vi "Setup.vi"(8 "error in (no error)":errorcluster, 11 "Mock Process Test In":refnum<class "Mock Process Test.lvclass">) -> (0 "error out":errorcluster, 3 "Mock Process Test Out":refnum<class "Mock Process Test.lvclass">)   [LabVIEW 2020, in "Mock Process Test.lvclass"]
uses:
  Base Class Test/Base Test.lvclass/Base Test.ctl
  Mock Process Test.lvclass
  Base Class Test/Base Test.lvclass
  Mock Process/Mock Process.lvclass
  C:/Users/anton/Documents/GitHub/Triarc-Framework/source/Framework/Process/Process.lvclass
  C:/Users/anton/Documents/GitHub/Triarc-Framework/source/Framework/Base/Base.lvclass
  C:/Users/anton/Documents/GitHub/Triarc-Framework/source/Framework/Error Handler Interface/Error Handler Interface.lvclass
  C:/Users/anton/Documents/GitHub/Triarc-Framework/source/Framework/Logging/Logging.lvclass
  C:/Users/anton/Documents/GitHub/Triarc-Framework/source/Framework Test/Mock Process/Mock Process.lvclass
  C:/Users/anton/Documents/GitHub/Triarc-Framework/source/Framework/Helper Loop/Helper Loop.lvclass
  C:/Users/anton/Documents/GitHub/Triarc-Framework/source/Framework Test/Process Test/Process Test.lvclass
  C:/Users/anton/Documents/GitHub/Triarc-Framework/source/Framework Test/Base Class Test/Base Test.lvclass
  C:/Program Files (x86)/National Instruments/LabVIEW 2020/vi.lib/Asteme/LUnit/Test Case.lvclass
  C:/Users/anton/Documents/GitHub/Triarc-Framework/source/Framework Test/Mock Process Test/Mock Process Test.lvclass
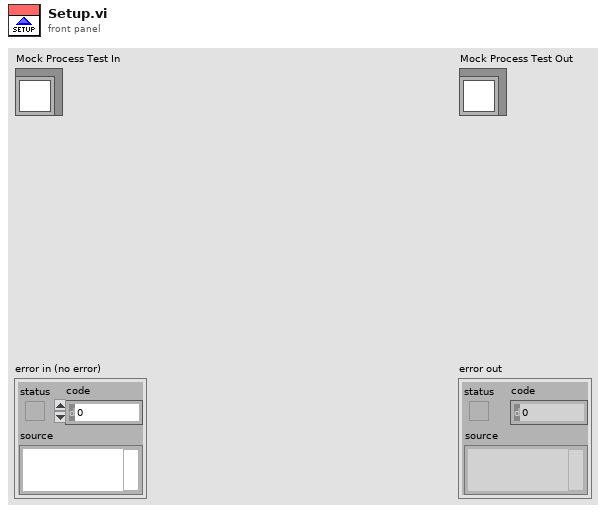
[diagram p1: front panel]
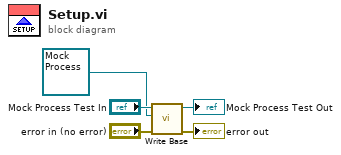
[diagram p0: block diagram]
diagram:
  n1 = call "Write Base.vi"("error in (no error)"="error in (no error)", "Base"=refnum<class "Mock Process.lvclass"> refnum ("Mock Process.lvclass"), "Base Class Test In"="Mock Process Test In") -> ("error out"=→"error out":errorcluster, "Base Class Test Out"=→"Mock Process Test Out":refnum<class "Mock Process Test.lvclass">)  [unwired: 7 in]
